vi "Process.vi"(8 "error in":errorcluster, 11 "Instrument UI in":refnum<class "Instrument UI.lvclass">) -> (0 "error out":errorcluster, 3 "Instrument UI out":refnum<class "Instrument UI.lvclass">)   [LabVIEW 2016, in "Instrument UI.lvclass"]
doc: "---------------------------------------------------------------\nJKI State Machine Objects™\nhttp://jki.net/state-machine-objects/\nCopyright (C) 2005-2015, JKI <info@jki.net>\nALL RIGHTS RESERVEDJKI State Machine Objects (SMO) 1.0.0.5\nJKI - JKI\nCopyright (c) 2016, JKI"
uses:
  Instrument UI.lvclass
  C:/Program Files (x86)/National Instruments/LabVIEW 2016/vi.lib/JKI/JKI SMO/SMO/SMO.lvclass
  C:/Program Files (x86)/National Instruments/LabVIEW 2016/vi.lib/JKI/JKI SMO/SMO.UI/SMO.UI.lvclass
  <vilib>/JKI/JKI SMO/SMO/Typedefs/Parent Call--Enum.ctl
  <vilib>/JKI/JKI SMO/SMO.UI/SMO.UI.lvclass
  <vilib>/JKI/JKI SMO/SMO/SMO.lvclass
panel:
  in  "STOP":bool
  # "Instrument UI.lvclass"
  # "For instructions on how to use the JKI State Machine Objects, examples and video tutorials, visit:\nhttp://jki.net/state-machine-objects/\n\nJKI State Machine Objects™\nhttp://jki.net/state-machine-objects/\nCopyright (C) 2005-2015, JKI <info@jki.net>\nALL RIGHTS RESERVED"
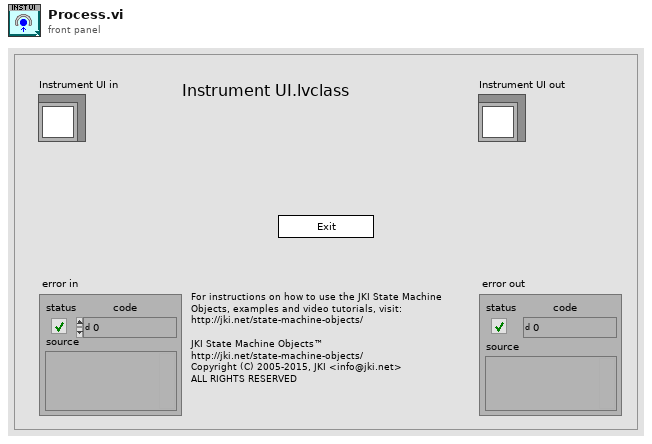
[diagram p1: front panel]
types:
  T1 = typedef "SMO.lvclass/Parent Call--Enum.ctl" = enum16{"Allows parent to run", "Does not request parent to run"}
  T2 = enum32{"invalid app kind", "Development System", "Run Time System", "Student Edition", "Embedded LabVIEW", "Evaluation", "Custom"}
  T3 = enum32{"Invalid", "Standard", "Closed", "Hidden", "Minimized", "Maximized"}
  T4 = cluster{"Core":cluster{"Current VI Reference":refnum<vi>, "Close Panel on Exit?":bool, "error":errorcluster}, "Self Reference":refnum<class "Instrument UI.lvclass">}
  T5 = cluster{"Current VI Reference":refnum<vi>, "Close Panel on Exit?":bool, "error":errorcluster}
  T6 = typedef "SMO.lvclass/Protected Events.ctl" = cluster{"StopProcesses":refnum<user-event>, "AbortProcesses":refnum<user-event>, "Config Changed":refnum<user-event>, "Dependency":refnum<user-event>}
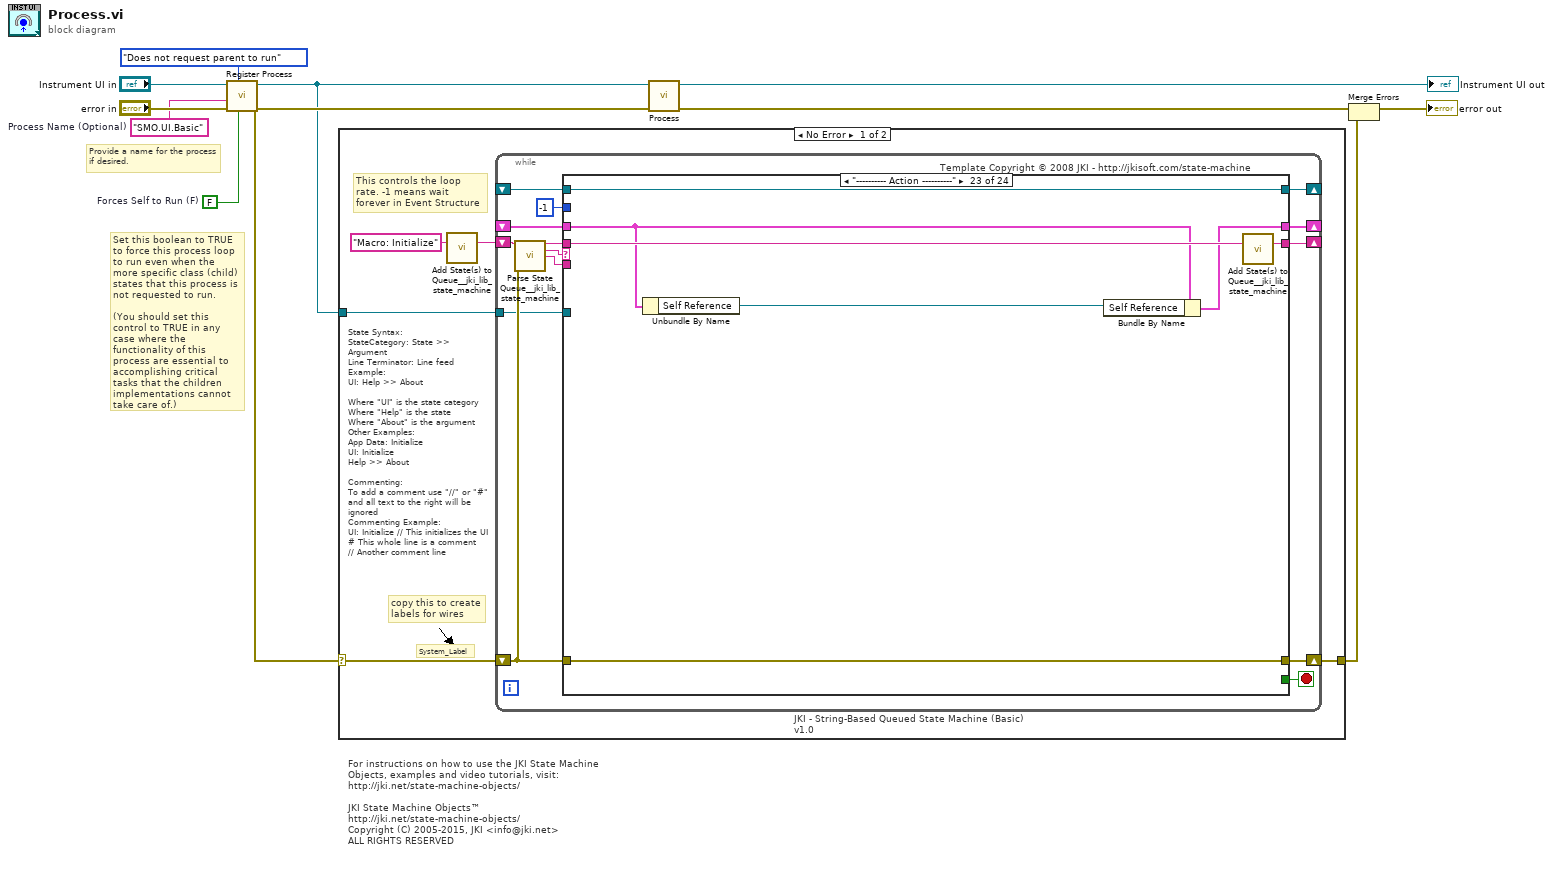
[diagram p0: block diagram]
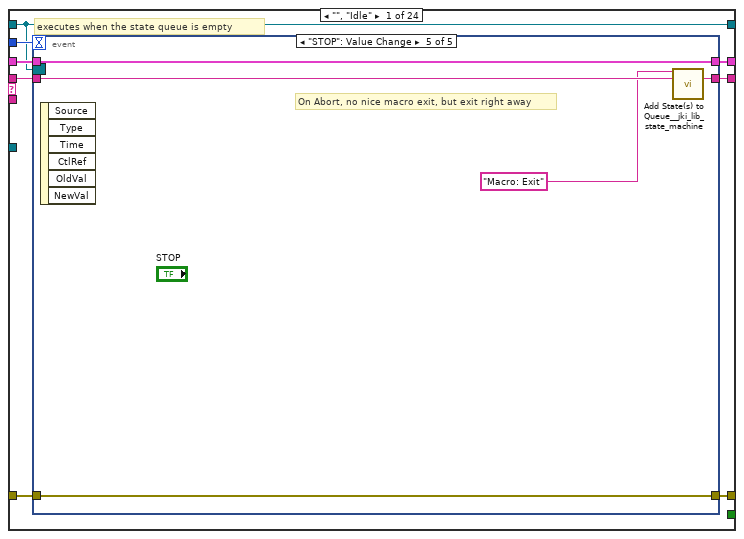
[diagram p2: hidden frame]
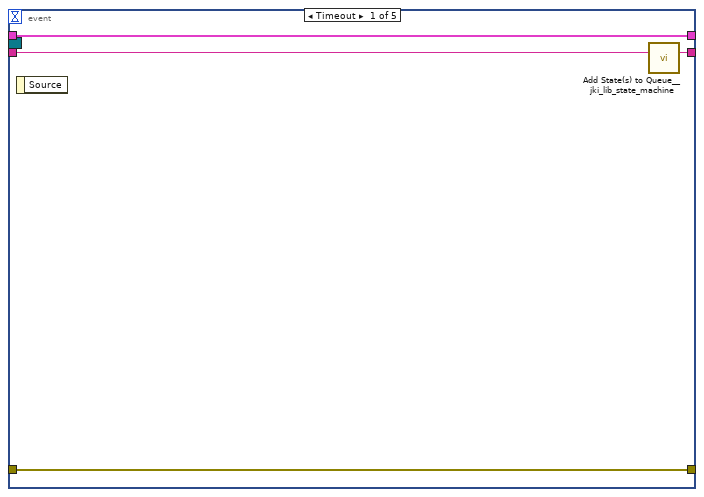
[diagram p3: hidden frame]
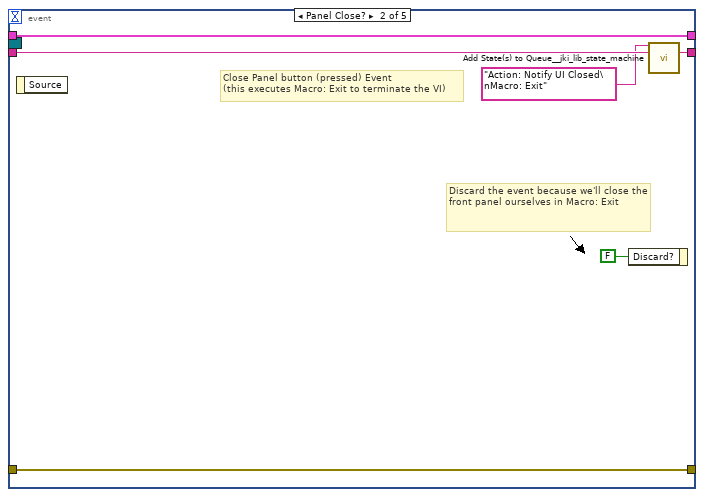
[diagram p4: hidden frame]
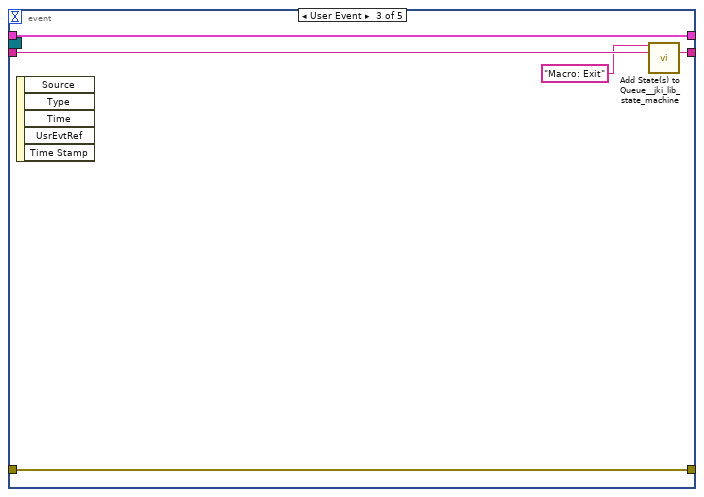
[diagram p5: hidden frame]
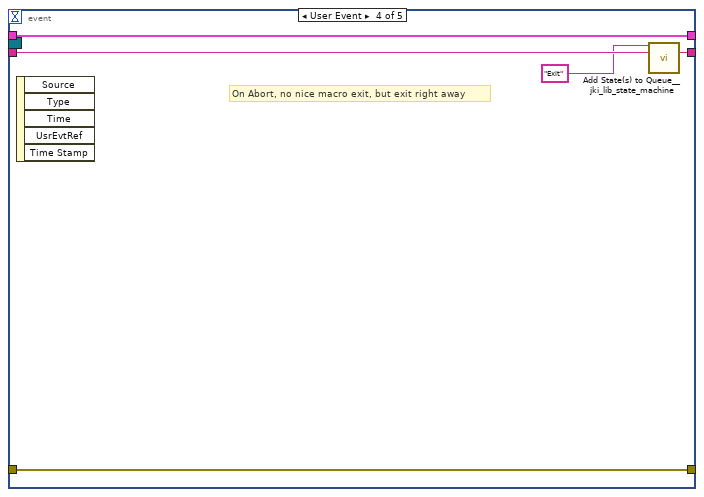
[diagram p6: hidden frame]
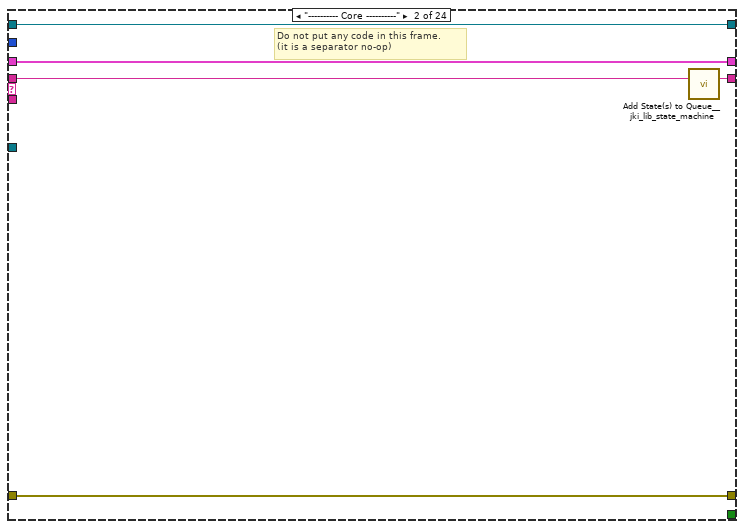
[diagram p7: hidden frame]
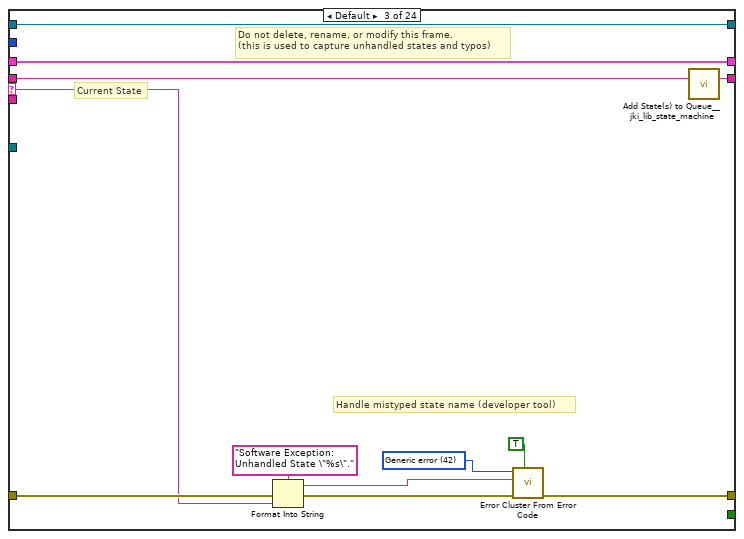
[diagram p8: hidden frame]
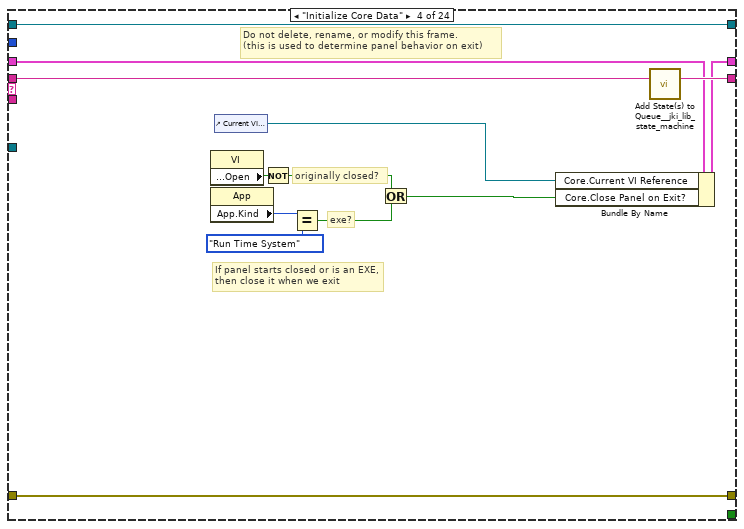
[diagram p9: hidden frame]
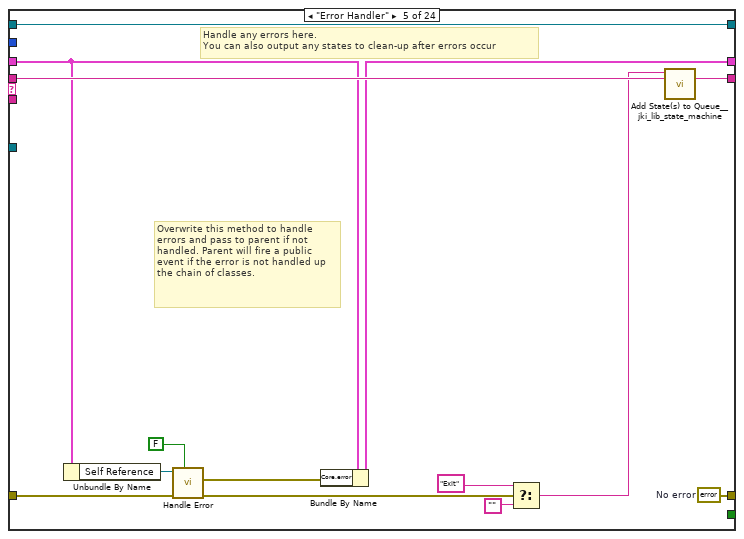
[diagram p10: hidden frame]
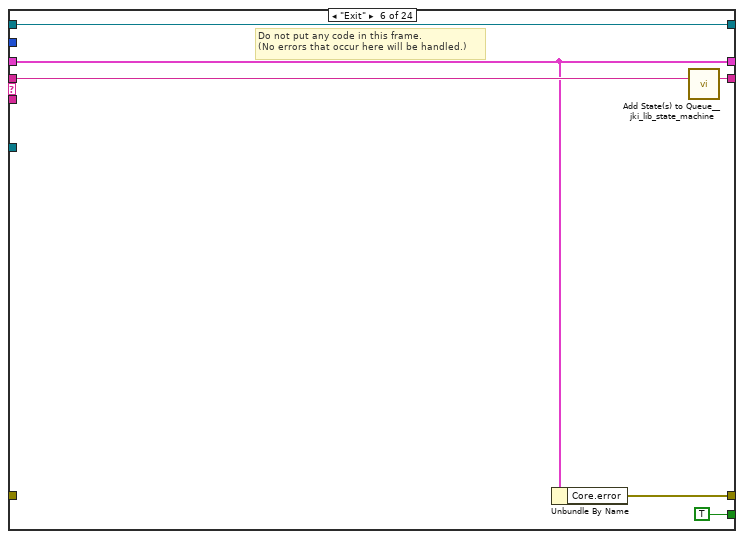
[diagram p11: hidden frame]
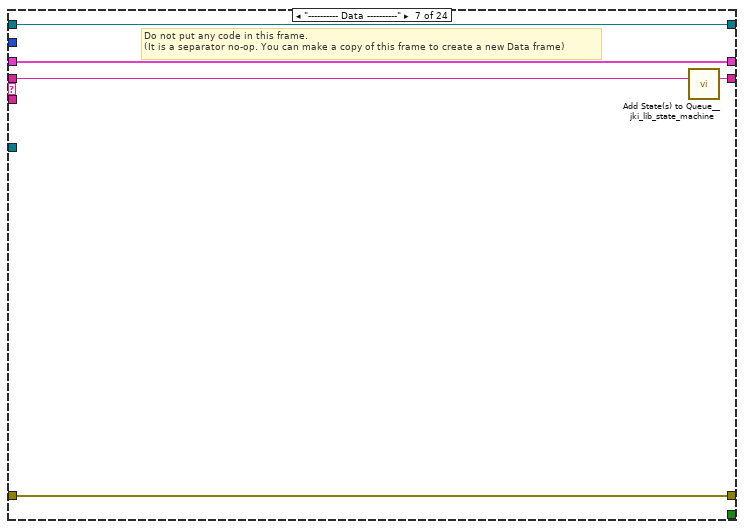
[diagram p12: hidden frame]
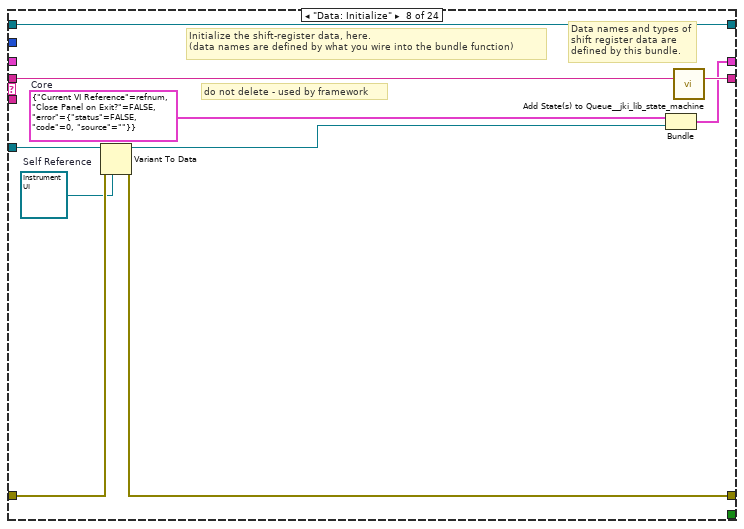
[diagram p13: hidden frame]
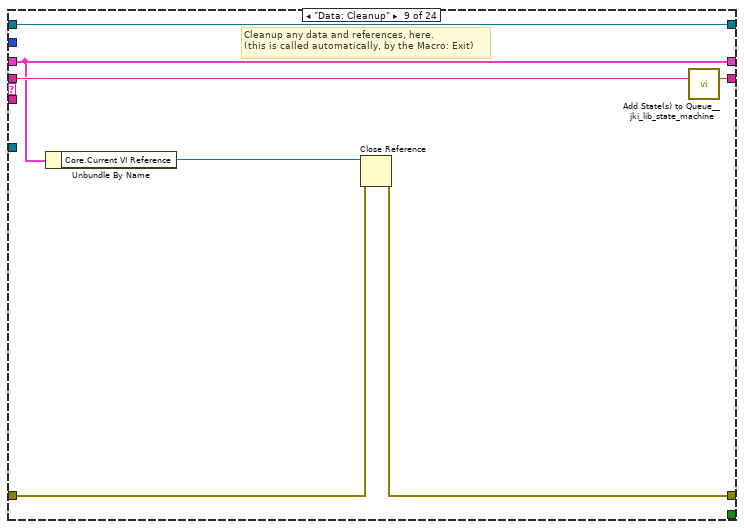
[diagram p14: hidden frame]
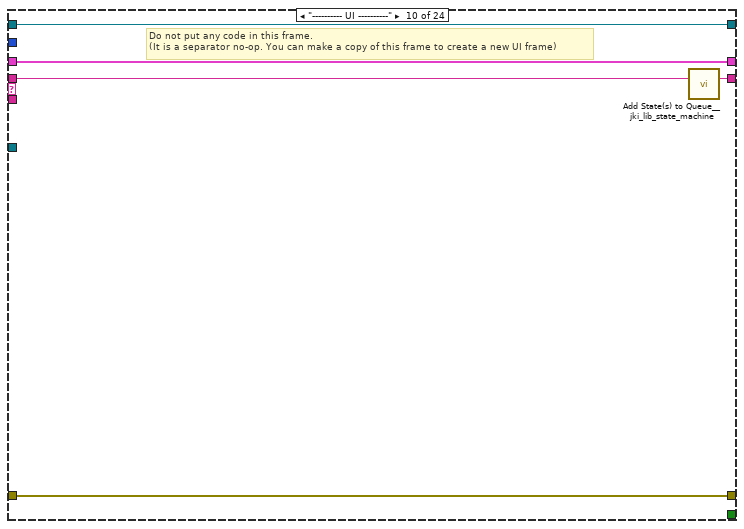
[diagram p15: hidden frame]
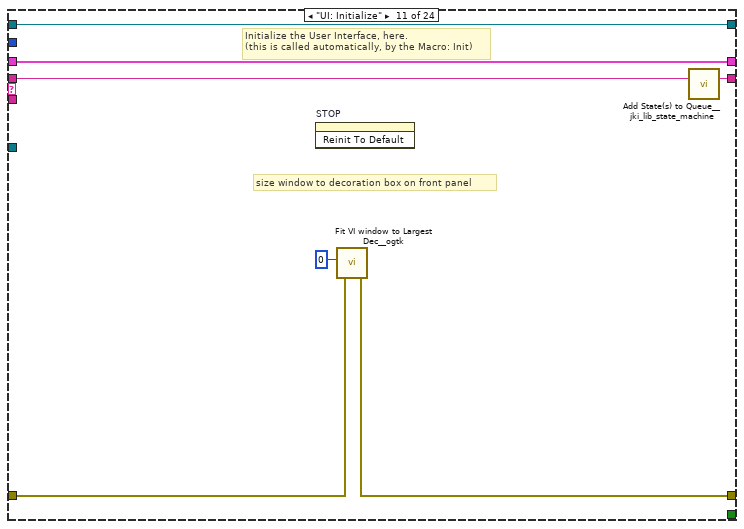
[diagram p16: hidden frame]
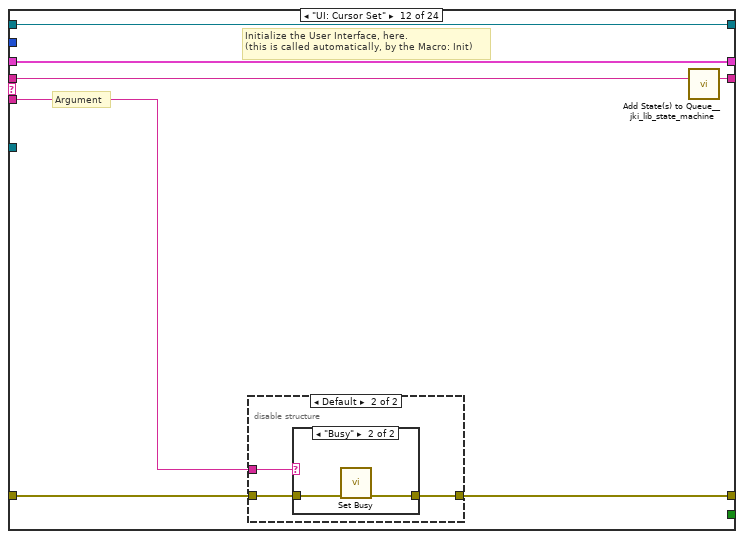
[diagram p17: hidden frame]
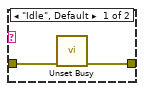
[diagram p19: hidden frame]
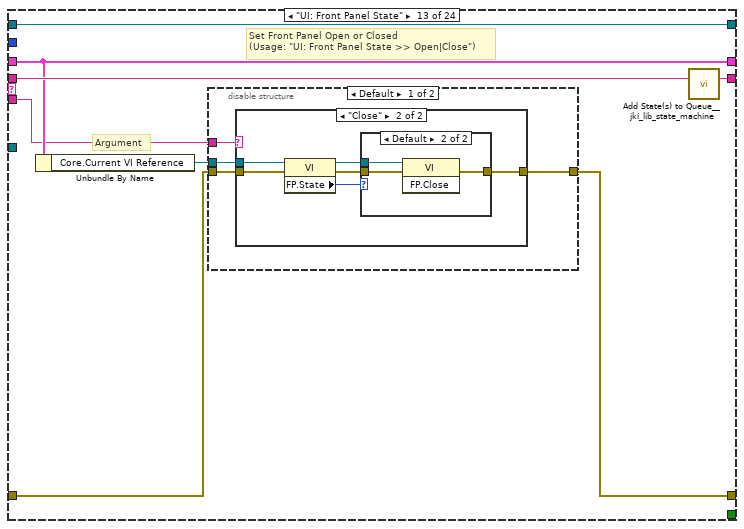
[diagram p20: hidden frame]
diagram:
  w2 = FALSE  # Forces Self to Run (F)
  w1 = "SMO.UI.Basic"  # Process Name (Optional)
  # "Provide a name for the process\nif desired."
  # "Set this boolean to TRUE to force this process loop to run even when the more specific class (child) states that this process is not requested to run.\n\n(You should set this control to TRUE in any case where the functionality of this process are essential to accomplishing critical tasks that the children implementations cannot take care of.)"
  # "For instructions on how to use the JKI State Machine Objects, examples and video tutorials, visit:\nhttp://jki.net/state-machine-objects/\n\nJKI State Machine Objects™\nhttp://jki.net/state-machine-objects/\nCopyright (C) 2005-2015, JKI <info@jki.net>\nALL RIGHTS RESERVED"
  n1 = call <vilib>:"Register Process.vi"("Forces Self to Run (F)"=w2, "Parent Call"=Parent_Call--Enum."Does not request parent to run", "error in (no error)"="error in", "Process Name (optional)"=w1, "SMO"="Instrument UI in") -> ("error out"=w8:errorcluster, "SMO out"=w7:refnum<class "Instrument UI.lvclass">)  [unwired: 5 in]
  n2 = case shown="No Error" w8 {
    selector: w8 -> [w13 w284]
    tunnel: w7 -> [w14 _]
    tunnel: [w12 w284] -> w4
    frame No Error {
      # "State Syntax:\nStateCategory: State >> Argument\nLine Terminator: Line feed\nExample:\nUI: Help >> About\n\nWhere \"UI\" is the state category\nWhere \"Help\" is the state\nWhere \"About\" is the argument\nOther Examples:\nApp Data: Initialize\nUI: Initialize\nHelp >> About\n\nCommenting:\nTo add a comment use \"//\" or \"#\" and all text to the right will be ignored\nCommenting Example:\nUI: Initialize // This initializes the UI\n# This whole line is a comment\n// Another comment line"
      # "copy this to create labels for wires"
      # "This controls the loop rate. -1 means wait forever in Event Structure"
      # "System_Label"
      n3 = call <vilib>:"Add State(s) to Queue__jki_lib_state_machine.vi"("State(s) in (\"\")"="Macro: Initialize") -> ("States Out"=w16:string)  [unwired: 14 in]
      n4 = while "JKI - String-Based Queued State Machine (Basic) v1.0" {
        shift-right: [w23] -> _
        shift-left: _ -> [w22]
        shift-right: [w26] -> w12
        shift-left: w13 -> [w20]
        shift-right: [w25] -> _
        shift-left: w16 -> [w27]
        tunnel: w14 -> [w19]
        shift-right: [w18] -> _
        shift-left: _ -> [w17]
        stop <- w24 stop-if-true
        # "Template Copyright © 2008 JKI - http://jkisoft.com/state-machine"
        n5 = call <vilib>:"Parse State Queue__jki_lib_state_machine.vi"("State Queue"=w27, "Error In (no error)"=w20) -> ("Remaining States"=w29:string, "Current State"=w30:string, "Arguments"=w28:string)  [unwired: 11 in]
        n6 = case shown="\"---------- Action ----------\"" w30 {
          selector: w30 -> [_ _ w70 _ _ _ _ _ _ _ _ _ _ _ _ _ _ _ _ _ _ _ _ _]
          tunnel: w29 -> [w38 w68 w74 w93 w107 w113 w118 w128 w135 w140 w147 w154 w170 w202 w211 w225 w230 w241 w248 w253 w263 w269 w276 w283]
          tunnel: w28 -> [_ _ _ _ _ _ _ _ _ _ _ w148 w164 _ _ _ _ _ _ _ _ _ _ _]
          tunnel: w22 -> [w36 w65 w72 w84 w96 w109 w115 _ w130 w137 w145 w152 w166 w199 w207 w216 w227 w238 w243 w250 w261 w267 w272 w279]
          tunnel: [w35 w66 w76 w90 w98 w108 w116 w120 w131 w138 w142 w149 w167 w200 w209 w223 w228 w232 w244 w251 w256 w264 w273 w277] -> w26
          tunnel: w20 -> [w34 w66 w75 w90 w103 _ w116 w125 w132 w138 w143 w150 w168 w200 w209 w223 w228 w233 w245 w251 w258 w265 w273 w278]
          tunnel: [w37 w67 w73 w92 w106 w112 w117 w127 w134 w139 w146 w153 w169 w201 w210 w224 w229 w240 w247 w252 w262 w268 w275 w282] -> w25
          tunnel: [_ _ _ _ _ TRUE _ _ _ _ _ _ _ _ _ _ _ _ _ _ _ _ _ _] -> w24
          tunnel: [w33 w65 w72 w91 w95 w109 w115 w126 w130 w137 w145 w152 w166 w199 w207 w216 w227 w238 w243 w250 w261 w267 w271 w279] -> w23
          tunnel: -1 ("Timeout") -> [w32 _ _ _ _ _ _ _ _ _ _ _ _ _ _ _ _ _ _ _ _ _ _ _]
          tunnel: w19 -> [_ _ _ _ _ _ _ w123 _ _ _ _ _ _ _ _ _ _ _ _ _ _ _ _]
          tunnel: [w31 w64 w69 w81 w105 w110 w114 w122 w129 w136 w144 w151 w163 w198 w208 w217 w226 w239 w246 w249 w260 w266 w274 w281] -> w18
          tunnel: w17 -> [w31 w64 w69 w81 w105 w110 w114 w122 w129 w136 w144 w151 w163 w198 w208 w217 w226 w239 w246 w249 _ w266 w274 w281]
          frame "", "Idle" {
            # "executes when the state queue is empty"
            n7 = event shown="[4] \"STOP\": Value Change" {
              selector: w31 -> [_ _ _ _ _]
              dyn-events: _ -> [_ _ _ _ _]
              timeout: w32 -> [_ _ _ _ _]
              tunnel: w38 -> [w42 w48 w53 w58 w63]
              tunnel: [w41 w47 w52 w57 w62] -> w37
              tunnel: w36 -> [w39 w44 w50 w55 w60]
              tunnel: [w40 w43 w51 w56 w61] -> w35
              tunnel: w34 -> [w40 w43 w51 w56 w61]
              tunnel: [w39 w44 w50 w55 w60] -> w33
              event Timeout {
                n8 = event-data() -> ()  [unwired: 1 in, 1 out]
                n9 = call <vilib>:"Add State(s) to Queue__jki_lib_state_machine.vi"("State(s) in (\"\")"=w42) -> ("States Out"=w41:string)  [unwired: 14 in]
              }
              event Panel Close? {
                # "Discard the event because we'll close the front panel ourselves in Macro: Exit"
                # "Close Panel button (pressed) Event\n(this executes Macro: Exit to terminate the VI)"
                n10 = event-data() -> ()  [unwired: 1 in, 1 out]
                n11 = event-data("Discard?"=FALSE) -> ()  [unwired: 1 in, 1 out]
                n12 = call <vilib>:"Add State(s) to Queue__jki_lib_state_machine.vi"("State(s) in Front (\"\")"="Action: Notify UI Closed\nMacro: Exit", "State(s) in (\"\")"=w48) -> ("States Out"=w47:string)  [unwired: 13 in]
              }
              event User Event {
                n13 = event-data() -> ()  [unwired: 1 in, 5 out]
                n14 = call <vilib>:"Add State(s) to Queue__jki_lib_state_machine.vi"("State(s) in Front (\"\")"="Macro: Exit", "State(s) in (\"\")"=w53) -> ("States Out"=w52:string)  [unwired: 13 in]
              }
              event User Event {
                # "On Abort, no nice macro exit, but exit right away"
                n15 = event-data() -> ()  [unwired: 1 in, 5 out]
                n16 = call <vilib>:"Add State(s) to Queue__jki_lib_state_machine.vi"("State(s) in Front (\"\")"="Exit", "State(s) in (\"\")"=w58) -> ("States Out"=w57:string)  [unwired: 13 in]
              }
              event "STOP": Value Change {
                # "On Abort, no nice macro exit, but exit right away"
                n17 = event-data() -> ()  [unwired: 1 in, 6 out]
                n18 = call <vilib>:"Add State(s) to Queue__jki_lib_state_machine.vi"("State(s) in Front (\"\")"="Macro: Exit", "State(s) in (\"\")"=w63) -> ("States Out"=w62:string)  [unwired: 13 in]
              }
            }
          }
          frame "---------- Core ----------" {
            # "Do not put any code in this frame.\n(it is a separator no-op)"
            n19 = call <vilib>:"Add State(s) to Queue__jki_lib_state_machine.vi"("State(s) in (\"\")"=w68) -> ("States Out"=w67:string)  [unwired: 14 in]
          }
          frame Default {
            w79 = 42 items=["No error", "Argument error", "Memory is full", "Out of zone", "End of file", "File already open", "Generic file I/O error", "File not found", "File permission error", "Disk is full", "Duplicate path", "Too many files open", "System feature not enabled", "Resource file not found", "Cannot add resource", "Resource not found", "Image not found", "Image memory error", "Pen does not exist", "Config type invalid", "Config token not found", "Config parse error", "Config memory error", "Bad external code format", "Bad external code offset", "External code not present", "Null window", "Destroy window error", "Null menu", "Print aborted", "Bad print record", "Print driver error", "Windows error during printing", "Memory error during printing", "Print dialog error", "Generic print error", "Invalid device refnum", "Device not found", "Device parameter error", "Device unit error", "Cannot open device", "Device call aborted", "Generic error", "Cancelled by user", "Object ID too low", "Object ID too high", "Object not in heap", "Unknown heap", "Unknown object (invalid DefProc)", "Unknown object (DefProc not in table)", "Message out of range", "Invalid (null) method", "Unknown message", "Manager call not supported", "Bad address", "Network operation in progress", "Network operation timed out", "Connection is busy", "Network attribute not supported", "Network error", "Address in use", "System out of memory", "Connection aborted", "Connection refused", "Not connected", "Already connected", "Connection closed", "Initialization error (interapplication manager)", "Bad occurrence", "Wait on unbound occurrence handler", "Occurrence queue overflow", "Datalog type conflict", "Unused", "Unrecognized type (interapplication manager)", "Memory corrupt", "Failed to make temporary DLL", "Old CIN version", "Drag socket not found", "Failed to load drop-object", "Failed to register OLE object", "Failed to release OLE object", "Format specifier type mismatch", "Unknown format specifier", "Too few format specifiers", "Too many format specifiers", "Scan failed", "Newer CIN version", "Error converting to variant", "Runtime menu error", "Password tampered", "Variant attribute not found", "Incompatible variant data type", "Event data is not available", "Event Store is not present", "Occurrence is not found", "Event Queue is not created", "Event info is not available", "Refnum passed is NULL", "Error retrieving Class GUID", "Error retrieving CoClass GUID", "Error retrieving TypeLib GUID.", "Bad built application magic bytes.", "Specific driver is different from the specific driver associated with the Logical Name.", "There is no session opened to the class driver.", "Max Error", "MAX - Error with config objects", "MAX - Error loading configuration", "MAX - Group not supported"]
            # "Current State"
            # "Do not delete, rename, or modify this frame.\n(this is used to capture unhandled states and typos)"
            # "Handle mistyped state name (developer tool)"
            n20 = Format Into String(format string="Software Exception: Unhandled State \"%s\"." ("message"), error in=w75, w70) -> (resulting string=w78:string, error out=w77:errorcluster)  [unwired: 1 in]
            n21 = call <vilib>:"Error Cluster From Error Code.vi"("show call chain? (False)"=TRUE, "error in (no error)"=w77, "error message (\"\")"=w78, "error code (0)"=w79) -> ("error out"=w76:errorcluster)  [unwired: 5 in]
            n22 = call <vilib>:"Add State(s) to Queue__jki_lib_state_machine.vi"("State(s) in (\"\")"=w74) -> ("States Out"=w73:string)  [unwired: 14 in]
          }
          frame "Initialize Core Data" {
            # "Do not delete, rename, or modify this frame.\n(this is used to determine panel behavior on exit)"
            # "originally closed?"
            # "exe?"
            # "If panel starts closed or is an EXE, then close it when we exit"
            n23 = property class="VI"() -> ("Front Panel.Open"=w89:bool)  [unwired: 2 in, 2 out]
            n24 = property class="App"() -> ("App.Kind"=w88:T2)  [unwired: 2 in, 2 out]
            n25 = control-ref of="Current VI Reference"() -> (w82:refnum<vi>)
            n26 = Not(x=w89) -> (.not. x?=w86:bool)
            n27 = Equal?(x=w88, y=T2."Run Time System" ("Application:Kind")) -> (x = y?=w85:bool)
            n28 = Or(x=w86, y=w85) -> (x .or. y?=w83:bool)
            n29 = Bundle By Name(cluster=w84, "Core.Current VI Reference"=w82, "Core.Close Panel on Exit?"=w83) -> (w91:T4)
            n30 = call <vilib>:"Add State(s) to Queue__jki_lib_state_machine.vi"("State(s) in (\"\")"=w93) -> ("States Out"=w92:string)  [unwired: 14 in]
          }
          frame "Error Handler" {
            w98 = errorcluster {"status"=FALSE, "code"=0, "source"=""}  # No error
            # "Overwrite this method to handle errors and pass to parent if not handled. Parent will fire a public event if the error is not handled up the chain of classes."
            # "Handle any errors here.\nYou can also output any states to clean-up after errors occur"
            n31 = Unbundle By Name(w96) -> ("Self Reference"=w104:refnum<class "Instrument UI.lvclass">)
            n32 = call-dynamic "Handle Error.vi"("Stop on Unhandled Error (T)"=FALSE, "error in"=w103, "Instrument UI"=w104) -> ("handling error"=w99:errorcluster, "Unhandled error"=w97:errorcluster)  [unwired: 6 in, 1 out]
            n33 = Bundle By Name(cluster=w96, "Core.error"=w97) -> (w95:T4)
            n34 = Select(t="Exit", s=w99, f="") -> (s? t:f=w100:string)
            n35 = call <vilib>:"Add State(s) to Queue__jki_lib_state_machine.vi"("State(s) in Front (\"\")"=w100, "State(s) in (\"\")"=w107) -> ("States Out"=w106:string)  [unwired: 13 in]
          }
          frame "Exit" {
            # "Do not put any code in this frame.\n(No errors that occur here will be handled.)"
            n36 = Unbundle By Name(w109) -> ("Core.error"=w108:errorcluster)
            n37 = call <vilib>:"Add State(s) to Queue__jki_lib_state_machine.vi"("State(s) in (\"\")"=w113) -> ("States Out"=w112:string)  [unwired: 14 in]
          }
          frame "---------- Data ----------" {
            # "Do not put any code in this frame.\n(It is a separator no-op. You can make a copy of this frame to create a new Data frame)"
            n38 = call <vilib>:"Add State(s) to Queue__jki_lib_state_machine.vi"("State(s) in (\"\")"=w118) -> ("States Out"=w117:string)  [unwired: 14 in]
          }
          frame "Data: Initialize" {
            w121 = T5 {"Current VI Reference"=refnum, "Close Panel on Exit?"=FALSE, "error"={"status"=FALSE, "code"=0, "source"=""}}  # Core
            w124 = refnum<class "Instrument UI.lvclass"> refnum  # Self Reference
            # "do not delete - used by framework"
            # "Data names and types of shift register data are defined by this bundle."
            # "Initialize the shift-register data, here.\n(data names are defined by what you wire into the bundle function)"
            n39 = Variant To Data(error in=w125, type=w124, Variant=w123) -> (data=w119:refnum<class "Instrument UI.lvclass">, error out=w120:errorcluster)
            n40 = Bundle("Core"=w121, "Self Reference"=w119) -> (w126:T4)  [unwired: 1 in]
            n41 = call <vilib>:"Add State(s) to Queue__jki_lib_state_machine.vi"("State(s) in (\"\")"=w128) -> ("States Out"=w127:string)  [unwired: 14 in]
          }
          frame "Data: Cleanup" {
            # "Cleanup any data and references, here.\n(this is called automatically, by the Macro: Exit)"
            n42 = Unbundle By Name(w130) -> ("Core.Current VI Reference"=w133:refnum<vi>)
            n43 = Close Reference(reference=w133, error in (no error)=w132) -> (error out=w131:errorcluster)
            n44 = call <vilib>:"Add State(s) to Queue__jki_lib_state_machine.vi"("State(s) in (\"\")"=w135) -> ("States Out"=w134:string)  [unwired: 14 in]
          }
          frame "---------- UI ----------" {
            # "Do not put any code in this frame.\n(It is a separator no-op. You can make a copy of this frame to create a new UI frame)"
            n45 = call <vilib>:"Add State(s) to Queue__jki_lib_state_machine.vi"("State(s) in (\"\")"=w140) -> ("States Out"=w139:string)  [unwired: 14 in]
          }
          frame "UI: Initialize" {
            # "size window to decoration box on front panel"
            # "Initialize the User Interface, here.\n(this is called automatically, by the Macro: Init)"
            n46 = invoke on="STOP" class="Bool (strict)" method="Reinit To Default"() -> ()  [unwired: 3 in, 3 out]
            n47 = call <userlib>:"Fit VI window to Largest Dec__ogtk.vi"("error in (no error)"=w143, "border spacing (2 px)"=0) -> ("error out"=w142:errorcluster)  [unwired: 4 in, 1 out]
            n48 = call <vilib>:"Add State(s) to Queue__jki_lib_state_machine.vi"("State(s) in (\"\")"=w147) -> ("States Out"=w146:string)  [unwired: 14 in]
          }
          frame "UI: Cursor Set" {
            # "Argument"
            # "Initialize the User Interface, here.\n(this is called automatically, by the Macro: Init)"
            n49 = disable-structure shown="Default" {
              disable-tunnel: w150 -> [w155 w158]
              disable-tunnel: [w155 w157] -> w149
              disable-tunnel: w148 -> [_ w156]
              frame condition #0 {
              }
              frame condition #1 (active) {
                n50 = case shown="\"Busy\"" w156 {
                  tunnel: w158 -> [w160 w162]
                  tunnel: [w159 w161] -> w157
                  frame "Idle", Default {
                    n51 = call <vilib>:"Unset Busy.vi"("error in (no error)"=w160) -> ("error out"=w159:errorcluster)  [unwired: 10 in]
                  }
                  frame "Busy" {
                    n52 = call <vilib>:"Set Busy.vi"("error in (no error)"=w162) -> ("error out"=w161:errorcluster)  [unwired: 9 in, 1 out]
                  }
                }
              }
            }
            n53 = call <vilib>:"Add State(s) to Queue__jki_lib_state_machine.vi"("State(s) in (\"\")"=w154) -> ("States Out"=w153:string)  [unwired: 14 in]
          }
          frame "UI: Front Panel State" {
            # "Argument"
            # "Set Front Panel Open or Closed\n(Usage: \"UI: Front Panel State >> Open|Close\")"
            n54 = Unbundle By Name(w166) -> ("Core.Current VI Reference"=w165:refnum<vi>)
            n55 = disable-structure shown="Default" {
              disable-tunnel: w168 -> [w174 w197]
              disable-tunnel: [w173 w197] -> w167
              disable-tunnel: w165 -> [w172 _]
              disable-tunnel: w164 -> [w171 _]
              frame condition #0 (active) {
                n56 = case shown="\"Close\"" w171 {
                  tunnel: w174 -> [w178 w191]
                  tunnel: [w180 w192] -> w173
                  tunnel: w172 -> [w179 w189]
                  frame "Open", Default {
                    n57 = property class="VI"(reference=w179, error in=w178) -> (reference out=w176:refnum<vi>, error out=w177:errorcluster, "FP.State"=w175:T3)
                    n58 = case shown="\"Closed\"" w175 {
                      tunnel: [w183 w186] -> w180
                      tunnel: w177 -> [w182 w186]
                      tunnel: w176 -> [w181 _]
                      frame "Closed" {
                        n59 = invoke class="VI" method="FP.Open"(reference=w181, error in=w182, "Activate"=TRUE, "State"=T3."Standard") -> (error out=w183:errorcluster)  [unwired: 1 in, 4 out]
                      }
                      frame Default {
                      }
                    }
                  }
                  frame "Close" {
                    n60 = property class="VI"(reference=w189, error in=w191) -> (reference out=w188:refnum<vi>, error out=w190:errorcluster, "FP.State"=w187:T3)
                    n61 = case shown="Default" w187 {
                      tunnel: [w193 w196] -> w192
                      tunnel: w190 -> [w193 w195]
                      tunnel: w188 -> [_ w194]
                      frame "Invalid", "Closed" {
                      }
                      frame Default {
                        n62 = invoke class="VI" method="FP.Close"(reference=w194, error in=w195) -> (error out=w196:errorcluster)  [unwired: 1 in, 2 out]
                      }
                    }
                  }
                }
              }
              frame condition #1 {
              }
            }
            n63 = call <vilib>:"Add State(s) to Queue__jki_lib_state_machine.vi"("State(s) in (\"\")"=w170) -> ("States Out"=w169:string)  [unwired: 14 in]
          }
          frame "---------- Macro ----------" {
            # "Do not put any code in this frame.\n(It is a separator no-op. You can make a copy of this frame to create a new Macro frame)"
            n64 = call <vilib>:"Add State(s) to Queue__jki_lib_state_machine.vi"("State(s) in (\"\")"=w202) -> ("States Out"=w201:string)  [unwired: 14 in]
          }
          frame "Macro: Initialize" {
            w205 = "UI: Initialize\n//UI: Front Panel State >> Open"  # UI: Initialize //UI: Front Panel State >> Open
            # "Initialization Macro\n(This is called once, when the VI starts)"
            n65 = call <vilib>:"Add State(s) to Queue__jki_lib_state_machine.vi"("State(s) in Front (\"\")"="Data: Initialize\nInitialize Core Data\nEvents: Register", "State(s) in (\"\")"="Process: Sync", "State(s) at Back (\"\")"=w205) -> ("States Out"=w204:string)  [unwired: 12 in]
            n66 = call <vilib>:"Add State(s) to Queue__jki_lib_state_machine.vi"("State(s) in Front (\"\")"=w204, "State(s) in (\"\")"=w211) -> ("States Out"=w210:string)  [unwired: 13 in]
          }
          frame "Macro: Exit" {
            # "Exit Macro\n(This is called once, when the VI exits)"
            n67 = Unbundle By Name(w216) -> ("Core.Close Panel on Exit?"=w222:bool)
            n68 = Select(t="UI: Front Panel State >> Close", s=w222, f="") -> (s? t:f=w219:string)
            n69 = call <vilib>:"Add State(s) to Queue__jki_lib_state_machine.vi"("State(s) in Front (\"\")"="Data: Cleanup\nEvents: Unregister\nProcess: Self Terminate", "State(s) in (\"\")"="Process: Sync", "State(s) at Back (\"\")"="Exit") -> ("States Out"=w213:string)  [unwired: 12 in]
            n70 = call <vilib>:"Add State(s) to Queue__jki_lib_state_machine.vi"("State(s) in (\"\")"=w219, "State(s) at Back (\"\")"=w213) -> ("States Out"=w218:string)  [unwired: 13 in]
            n71 = call <vilib>:"Add State(s) to Queue__jki_lib_state_machine.vi"("State(s) in Front (\"\")"=w218, "State(s) in (\"\")"=w225) -> ("States Out"=w224:string)  [unwired: 13 in]
          }
          frame "---------- Process ----------" {
            # "Template Separator\n(You can make a copy of, or modify, this frame)"
            n72 = call <vilib>:"Add State(s) to Queue__jki_lib_state_machine.vi"("State(s) in (\"\")"=w230) -> ("States Out"=w229:string)  [unwired: 14 in]
          }
          frame "Process: Sync" {
            n73 = Unbundle By Name(w238) -> ("Self Reference"=w234:refnum<class "Instrument UI.lvclass">)
            n74 = call <vilib>:"WaitOnProcessSync.vi"("error in (no error)"=w233, "SMO"=w234) -> ("error out"=w232:errorcluster, "Don't run?"=w237:bool)  [unwired: 7 in, 1 out]
            n75 = Select(t="Data: Cleanup\nEvents: Unregister\nExit", s=w237, f="") -> (s? t:f=w231:string)
            n76 = call <vilib>:"Add State(s) to Queue__jki_lib_state_machine.vi"("State(s) in Front (\"\")"=w231, "State(s) in (\"\")"=w241) -> ("States Out"=w240:string)  [unwired: 13 in]
          }
          frame "Process: Self Terminate" {
            n77 = Unbundle By Name(w243) -> ("Self Reference"=w242:refnum<class "Instrument UI.lvclass">)
            n78 = call <vilib>:"SelfTerminate.vi"("error in (no error)"=w245, "SMO in"=w242) -> ("error out"=w244:errorcluster)  [unwired: 8 in, 1 out]
            n79 = call <vilib>:"Add State(s) to Queue__jki_lib_state_machine.vi"("State(s) in (\"\")"=w248) -> ("States Out"=w247:string)  [unwired: 14 in]
          }
          frame "---------- Events ----------" {
            # "Template Separator\n(You can make a copy of, or modify, this frame)"
            n80 = call <vilib>:"Add State(s) to Queue__jki_lib_state_machine.vi"("State(s) in (\"\")"=w253) -> ("States Out"=w252:string)  [unwired: 14 in]
          }
          frame "Events: Register" {
            # "Expand to add\nmore events"
            # "Base Class Protected Events"
            n81 = Unbundle By Name(w261) -> ("Self Reference"=w254:refnum<class "Instrument UI.lvclass">)
            n82 = call <vilib>:"GetProtectedEvents.vi"("SMO"=w254) -> ("error out"=w255:errorcluster, "SMO Protected Events"=w259:T6)  [unwired: 8 in, 1 out]
            n83 = register-events(w259) -> (reference out=w260:refnum<event-registration>, error out=w257:errorcluster)  [unwired: 2 in]
            n84 = Merge Errors(w258, w257, w255) -> (w256:errorcluster)
            n85 = call <vilib>:"Add State(s) to Queue__jki_lib_state_machine.vi"("State(s) in (\"\")"=w263) -> ("States Out"=w262:string)  [unwired: 14 in]
          }
          frame "Events: Unregister" {
            n86 = Unregister For Events(event registration refnum=w266, error in=w265) -> (error out=w264:errorcluster)
            n87 = call <vilib>:"Add State(s) to Queue__jki_lib_state_machine.vi"("State(s) in (\"\")"=w269) -> ("States Out"=w268:string)  [unwired: 14 in]
          }
          frame "---------- Action ----------" {
            n88 = Unbundle By Name(w272) -> ("Self Reference"=w270:refnum<class "Instrument UI.lvclass">)
            n89 = Bundle By Name(cluster=w272, "Self Reference"=w270) -> (w271:T4)
            n90 = call <vilib>:"Add State(s) to Queue__jki_lib_state_machine.vi"("State(s) in (\"\")"=w276) -> ("States Out"=w275:string)  [unwired: 14 in]
          }
          frame "Action: Notify UI Closed" {
            # "Notify that the UI has been closed"
            n91 = Unbundle By Name(w279) -> ("Self Reference"=w280:refnum<class "Instrument UI.lvclass">)
            n92 = call <vilib>:"Hide.vi"("error in (no error)"=w278, "SMO.UI"=w280) -> ("error out"=w277:errorcluster)  [unwired: 8 in, 1 out]
            n93 = call <vilib>:"Add State(s) to Queue__jki_lib_state_machine.vi"("State(s) in (\"\")"=w283) -> ("States Out"=w282:string)  [unwired: 14 in]
          }
        }
      }
    }
    frame Error {
    }
  }
  n94 = call-parent "Process.vi"("error in (no error)"=w8, "SMO.UI"=w7) -> ("error out"=w5:errorcluster, "SMO.UI out"=→"Instrument UI out":refnum<class "Instrument UI.lvclass">)  [unwired: 8 in]
  n95 = Merge Errors(w5, w4) -> (→"error out":errorcluster)
